vi "deltaArray.vi"(1 "Array":dbl[][](array[numeric])) -> (0 "Delta Array":dbl[][](array[numeric]))   [LabVIEW 2017]
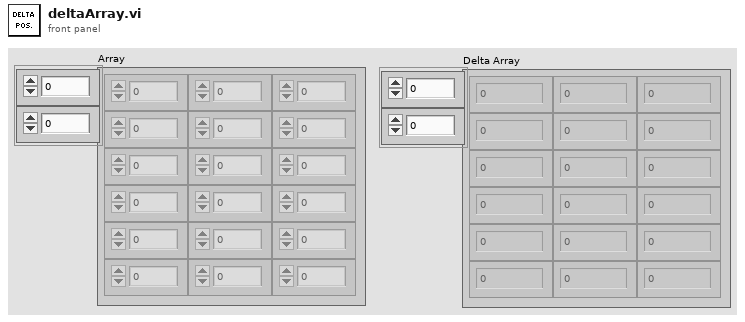
[diagram p1: front panel]
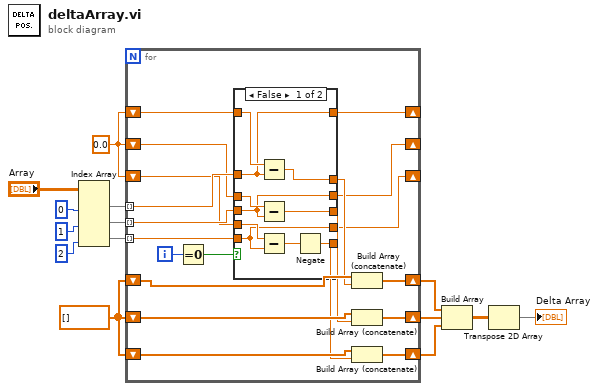
[diagram p0: block diagram]
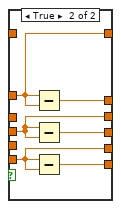
[diagram p2: hidden frame]
diagram:
  w2 = 0.0
  w1 = dbl[] []
  n1 = Index Array(array="Array", index (col) #1=0 ("disabled index (col)"), index (col) #2=1 ("index (col)"), index (col) #3=2 ("index (col)")) -> (element #1=w10:dbl[], element #2=w9:dbl[], element #3=w8:dbl[])  [unwired: 3 in]
  n2 = for {
    tunnel: w10 -> [w30] mode=indexing
    tunnel: w9 -> [w29] mode=indexing
    tunnel: w8 -> [w28] mode=indexing
    shift-right: [w34] -> w7
    shift-left: w1 -> [w26]
    shift-right: [w33] -> w6
    shift-left: w1 -> [w27]
    shift-right: [w32] -> w5
    shift-left: w1 -> [w25]
    shift-right: [w17] -> _
    shift-left: w2 -> [w22]
    shift-right: [w16] -> _
    shift-left: w2 -> [w20]
    shift-right: [w15] -> _
    shift-left: w2 -> [w18]
    i -> [w24]
    n3 = Equal To 0?(x=w24) -> (x = 0?=w31:bool)
    n4 = case shown="False" w31 {
      tunnel: [w35 w50] -> w19
      tunnel: [w43 w49] -> w21
      tunnel: [w44 w48] -> w23
      tunnel: w30 -> [w39 w47]
      tunnel: w29 -> [w38 w46]
      tunnel: w28 -> [w37 w45]
      tunnel: w22 -> [w42 _]
      tunnel: w20 -> [w41 _]
      tunnel: w18 -> [w40 _]
      tunnel: [w39 w47] -> w17
      tunnel: [w38 w46] -> w16
      tunnel: [w37 w45] -> w15
      frame False {
        n5 = Subtract(x=w42, y=w39) -> (x-y=w44:dbl)
        n6 = Subtract(x=w41, y=w38) -> (x-y=w43:dbl)
        n7 = Subtract(x=w40, y=w37) -> (x-y=w36:dbl)
        n8 = Negate(x=w36) -> (-x=w35:dbl)
      }
      frame True {
        n9 = Subtract(x=w47, y=w47) -> (x-y=w48:dbl)
        n10 = Subtract(x=w46, y=w46) -> (x-y=w49:dbl)
        n11 = Subtract(x=w45, y=w45) -> (x-y=w50:dbl)
      }
    }
    n12 = Build Array (concatenate)(w26, w23) -> (w34:dbl[])
    n13 = Build Array (concatenate)(w27, w21) -> (w33:dbl[])
    n14 = Build Array (concatenate)(w25, w19) -> (w32:dbl[])
  }
  n15 = Build Array(w7, w6, w5) -> (w3:dbl[][])
  n16 = Transpose 2D Array(2D array=w3) -> (transposed array=→"Delta Array":dbl[][])
